vi "Target - REF - MAIN.vi"() -> ()   [LabVIEW 2013]
doc: "This VI first configures the sample clock on the module and starts it. Then it acquires single point data from four channels. In order for the loop rate to be synchronized with the module's clock, the data is pipelined before it is written it to a DMA FIFO so it can be transfered to the host."
uses:
  <vilib>/LabVIEW Targets/FPGA/cRIO/shared/nicrio_ModuleControls/nicrio_cRIO-9234_DataRatesRing2.ctl
  <vilib>/rvi/eio/common/nirviEmuTemplatePropertySet_errors.vi
  <vilib>/rvi/eio/common/nirviEmuTemplateMethod_errors.vi
  <vilib>/rvi/Emulation/niFpgaSctlEmulationGetInTimedLoop.vi
  <vilib>/rvi/Emulation/niFpgaEmulationReportErrorSimple.vi
  <vilib>/rvi/Emulation/niFpgaGetClockAttributes.vi
  <vilib>/rvi/Emulation/niFpgaCriticalErrorInLSC.vi
  <vilib>/rvi/eio/common/nirviEmuTemplatePropertyGet_noerrors.vi
  <vilib>/rvi/interface/RandomDataEmulation/nirviRandomDataFPGAFIFO.vi
  <vilib>/rvi/interface/RandomDataEmulation/niFpgaRandomDataHandleErrors.vi
  <vilib>/eio/EIOPropertyNode/EIOPropertyNode.xnode
  <vilib>/eio/EIONode/EIONode.xnode
  <vilib>/eio/EIOMethodNode/EIOMethodNode.xnode
  <vilib>/rvi/DataTransferAndStorage/Container/XNode/niFpgaContainer.xnode
  <vilib>/rvi/interface/RandomDataEmulation/nirviRandomDataFpgaReadWriteTemplate.vi
  <vilib>/rvi/eio/common/nirviEmuTemplatePropertyGet_errors.vi
  <vilib>/rvi/eio/common/nirviEmuTemplatePropertySet_noerrors.vi
  GPS Timekeeper Files/FPGA Timekeeper.lvlib
panel:
  out "FPGA Timekeeper time (ns)":u64
  out "GPS status":T1(ring)
  out "FPGA Timekeeper locked":bool
  out "offset from time reference":i32
  out "antenna status":T2(ring)
  out "satellites available":u8
  out "UTC offset":i8
  out "UTC offset valid":bool
  in  "Data Rate":T3=1 items=["51.200 kS/s (NI 9234)"=1, "25.600 kS/s (NI 9234)"=2, "17.067 kS/s (NI 9234)"=3, "12.800 kS/s (NI 9234)"=4, "10.240 kS/s (NI 9234)"=5, "8.533 kS/s (NI 9234)"=6, "7.314 kS/s (NI 9234)"=7, "6.400 kS/s (NI 9234)"=8, "5.689 kS/s (NI 9234)"=9, "5.120 kS/s (NI 9234)"=10, "4.654 kS/s (NI 9234)"=11, "4.267 kS/s (NI 9234)"=12, "3.938 kS/s (NI 9234)"=13, "3.657 kS/s (NI 9234)"=14, "3.413 kS/s (NI 9234)"=15, "3.200 kS/s (NI 9234)"=16, "3.012 kS/s (NI 9234)"=17, "2.845 kS/s (NI 9234)"=18, "2.695 kS/s (NI 9234)"=19, "2.560 kS/s (NI 9234)"=20, "2.438 kS/s (NI 9234)"=21, "2.328 kS/s (NI 9234)"=22, "2.226 kS/s (NI 9234)"=23, "2.133 kS/s (NI 9234)"=24, "2.048 kS/s (NI 9234)"=25, "1.969 kS/s (NI 9234)"=26, "1.896 kS/s (NI 9234)"=27, "1.829 kS/s (NI 9234)"=28, "1.765 kS/s (NI 9234)"=29, "1.707 kS/s (NI 9234)"=30, "1.652 kS/s (NI 9234)"=31]
  out "Acq Loop Ticks":u32
  out "FPGA Error":errorcluster
  out "Module Underflow":bool
  out "DMA FIFO Full":bool
  in  "Stop":bool
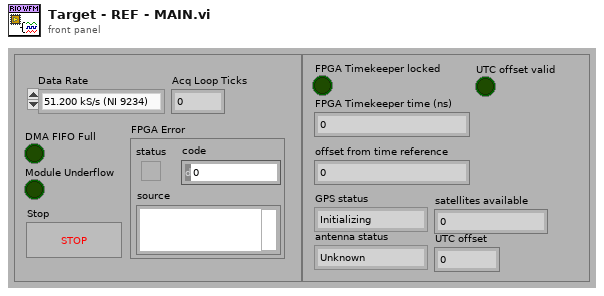
[diagram p1: front panel]
types:
  T1 = enum8{"Initializing", "Normal", "Unable to get fix"}
  T2 = enum8{"Unknown", "Normal", "Absent", "Overcurrent"}
  T3 = typedef "nicrio_cRIO-9234_DataRatesRing2.ctl" = u8
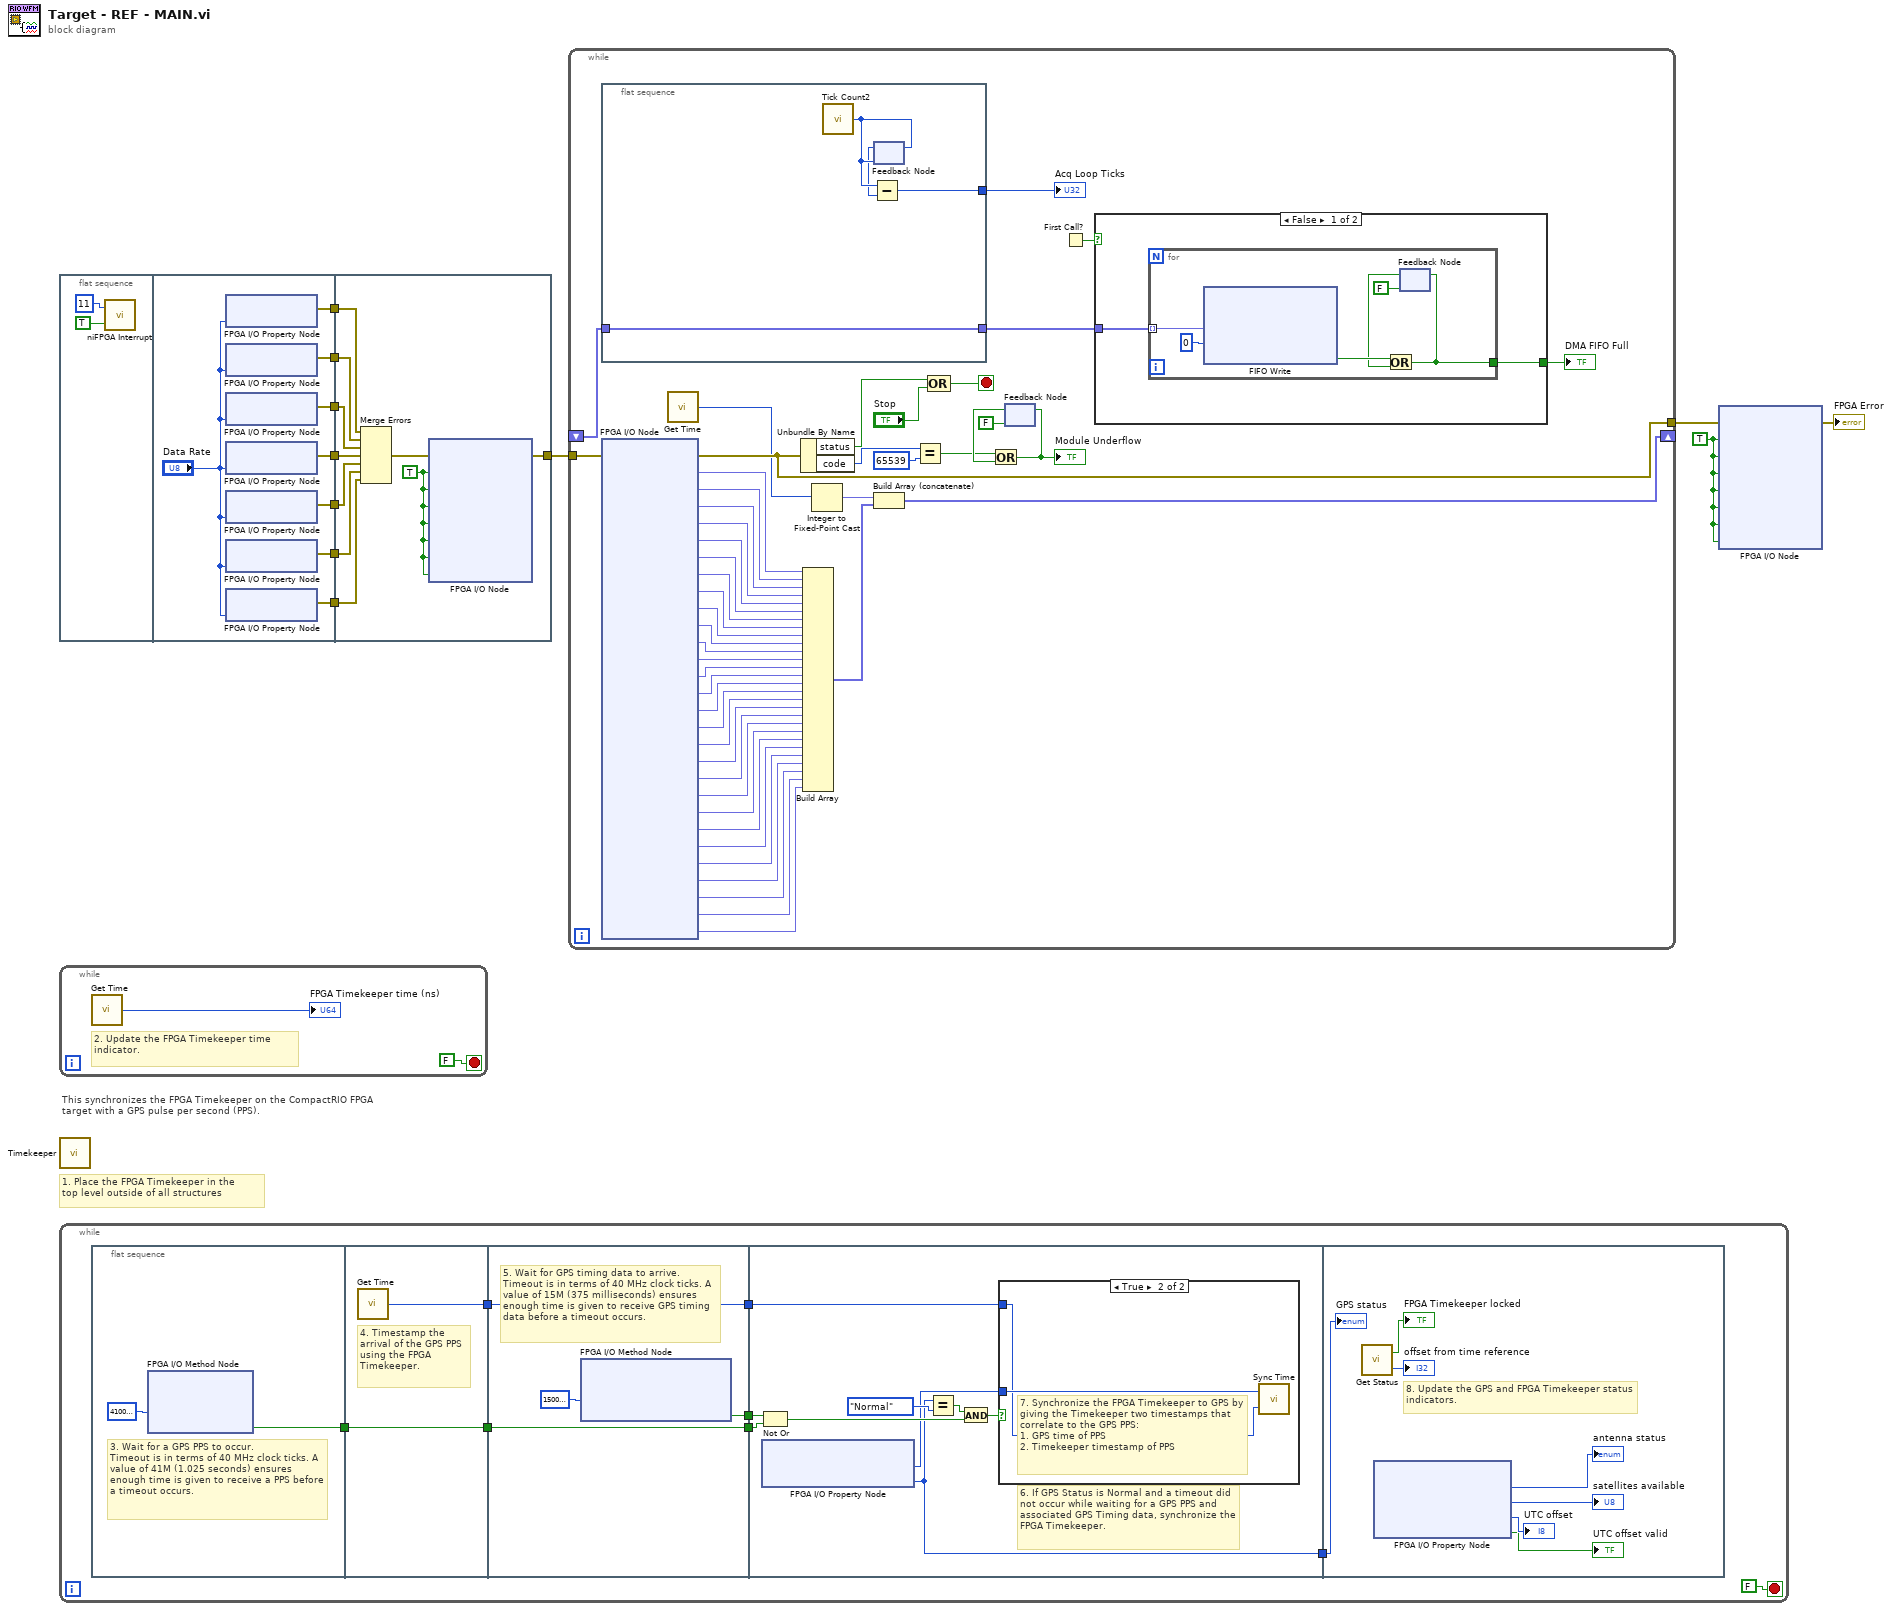
[diagram p0: block diagram]
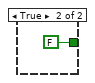
[diagram p3: hidden frame]
diagram:
  w1 = TRUE ("Mod1/Stop")
  # "This synchronizes the FPGA Timekeeper on the CompactRIO FPGA target with a GPS pulse per second (PPS)."
  # "1. Place the FPGA Timekeeper in the\ntop level outside of all structures"
  n1 = flat-sequence {
    tunnel: [w21] -> w10
    tunnel: [w20] -> w9
    tunnel: [w19] -> w6
    tunnel: [w18] -> w5
    tunnel: [w16] -> w4
    tunnel: [w15] -> w3
    tunnel: [w14] -> w2
    tunnel: [w31] -> w11
    tunnel: w10 -> [w29]
    tunnel: w9 -> [w28]
    tunnel: w6 -> [w27]
    tunnel: w5 -> [w26]
    tunnel: w4 -> [w25]
    tunnel: w3 -> [w24]
    tunnel: w2 -> [w23]
    frame #0 {
      n2 = call <vilib>:"niFPGA Interrupt.vi"("Wait Until Cleared (F)"=TRUE ("Wait Until Cleared"), "IRQ Number (0)"=u8 11 ("IRQ Number")) -> ()  [unwired: 1 in]
    }
    frame #1 {
      n3 = xnode "FPGA I/O Property Node"("Data Rate"="Data Rate") -> ("error out"=w21:errorcluster)  [unwired: 2 in, 1 out]
      n4 = xnode "FPGA I/O Property Node"("Data Rate"="Data Rate") -> ("error out"=w20:errorcluster)  [unwired: 2 in, 1 out]
      n5 = xnode "FPGA I/O Property Node"("Data Rate"="Data Rate") -> ("error out"=w19:errorcluster)  [unwired: 2 in, 1 out]
      n6 = xnode "FPGA I/O Property Node"("Data Rate"="Data Rate") -> ("error out"=w18:errorcluster)  [unwired: 2 in, 1 out]
      n7 = xnode "FPGA I/O Property Node"("Data Rate"="Data Rate") -> ("error out"=w16:errorcluster)  [unwired: 2 in, 1 out]
      n8 = xnode "FPGA I/O Property Node"("Data Rate"="Data Rate") -> ("error out"=w15:errorcluster)  [unwired: 2 in, 1 out]
      n9 = xnode "FPGA I/O Property Node"("Data Rate"="Data Rate") -> ("error out"=w14:errorcluster)  [unwired: 2 in, 1 out]
    }
    frame #2 {
      w22 = TRUE ("Mod1/Start")
      n10 = Merge Errors(w29, w28, w27, w26, w25, w24, w23) -> (w30:errorcluster)
      n11 = xnode "FPGA I/O Node"("error in"=w30, "Mod1/Start"=w22, "Mod2/Start"=w22, "Mod3/Start"=w22, "Mod4/Start"=w22, "Mod5/Start"=w22, "Mod6/Start"=w22, "Mod7/Start"=w22) -> ("error out"=w31:errorcluster)  [unwired: 7 in, 7 out]
    }
  }
  n12 = while {
    stop <- FALSE stop-if-true
    # "2. Update the FPGA Timekeeper time indicator."
    n13 = call "Get Time.vi"() -> ("time (ns)"=→"FPGA Timekeeper time (ns)":u64)  [unwired: 1 in]
  }
  n14 = call "Timekeeper.vi"() -> ()  [unwired: 12 in]
  n15 = while {
    stop <- FALSE stop-if-true
    n16 = flat-sequence {
      tunnel: [w42] -> w40
      tunnel: w40 -> [w45]
      tunnel: [w45] -> w39
      tunnel: [w44] -> w37
      tunnel: [w48] -> w41
      tunnel: w39 -> [w47]
      tunnel: [w47] -> w38
      tunnel: w37 -> [w46]
      tunnel: [w46] -> w36
      tunnel: w41 -> [w57]
      tunnel: w38 -> [w56]
      tunnel: w36 -> [w51]
      tunnel: [w50] -> w35
      tunnel: w35 -> [w67]
      frame #0 {
        # "3. Wait for a GPS PPS to occur.\nTimeout is in terms of 40 MHz clock ticks. A value of 41M (1.025 seconds) ensures enough time is given to receive a PPS before a timeout occurs."
        n17 = xnode "FPGA I/O Method Node"("Timeout"=41000000) -> ("Timed Out"=w42:bool)  [unwired: 1 in, 1 out]
      }
      frame #1 {
        # "4. Timestamp the arrival of the GPS PPS using the FPGA Timekeeper."
        n18 = call "Get Time.vi"() -> ("time (ns)"=w44:u64)  [unwired: 1 in]
      }
      frame #2 {
        # "5. Wait for GPS timing data to arrive.\nTimeout is in terms of 40 MHz clock ticks. A value of 15M (375 milliseconds) ensures enough time is given to receive GPS timing data before a timeout occurs."
        n19 = xnode "FPGA I/O Method Node"("Timeout"=15000000) -> ("Timed Out"=w48:bool)  [unwired: 1 in, 1 out]
      }
      frame #3 {
        # "6. If GPS Status is Normal and a timeout did not occur while waiting for a GPS PPS and associated GPS Timing data, synchronize the FPGA Timekeeper."
        n20 = Not Or(1:w56, 2:w57) -> (0:w54:bool)
        n21 = xnode "FPGA I/O Property Node"() -> ("PPS Timestamp (TAI)"=w52:u64, "GPS Status"=w50:T1)  [unwired: 1 in, 1 out]
        n22 = Equal?(x=w50, y=T1."Normal") -> (x = y?=w55:bool)
        n23 = And(x=w55, y=w54) -> (x .and. y?=w53:bool)
        n24 = case shown="True" w53 {
          tunnel: w52 -> [_ w60]
          tunnel: w51 -> [_ w59]
          frame False {
          }
          frame True {
            # "7. Synchronize the FPGA Timekeeper to GPS by giving the Timekeeper two timestamps that correlate to the GPS PPS:\n1. GPS time of PPS\n2. Timekeeper timestamp of PPS"
            n25 = call "Sync Time.vi"("FPGA Timekeeper time (ns)"=w59, "time reference time (ns)"=w60) -> ()
          }
        }
      }
      frame #4 {
        # "8. Update the GPS and FPGA Timekeeper status indicators."
        n26 = call "Get Status.vi"() -> ("FPGA Timekeeper locked"=→"FPGA Timekeeper locked":bool, "offset from time reference"=→"offset from time reference":i32)
        n27 = xnode "FPGA I/O Property Node"() -> ("Antenna Status"=→"antenna status":T2, "Satellites Available"=→"satellites available":u8, "UTC Offset"=→"UTC offset":i8, "UTC Offset Valid"=→"UTC offset valid":bool)  [unwired: 1 in, 1 out]
        "GPS status" <- w67
      }
    }
  }
  n28 = while {
    tunnel: [w111] -> w8
    shift-right: [w99] -> _
    shift-left: _ -> [w107]
    tunnel: w11 -> [w100]
    stop <- w114 stop-if-true
    n29 = flat-sequence {
      tunnel: [w126] -> w109
      tunnel: w107 -> [w125]
      tunnel: [w125] -> w108
      frame #0 {
        n30 = call "Tick Count2"() -> ("Tick Count(Ticks)"=w128:u32)
        n31 = feedback-in #1(w128) -> ()
        n32 = feedback #1(w128) -> (w127:u32)
        n33 = Subtract(x=w128, y=w127) -> (x-y=w126:u32)
      }
    }
    n34 = xnode "FPGA I/O Node"("error in"=w100) -> ("error out"=w111:errorcluster, "Mod1/AI0"=w96:fxp<+/-,24,4>, "Mod1/AI1"=w95:fxp<+/-,24,4>, "Mod1/AI2"=w94:fxp<+/-,24,4>, "Mod1/AI3"=w93:fxp<+/-,24,4>, "Mod2/AI0"=w92:fxp<+/-,24,4>, "Mod2/AI1"=w91:fxp<+/-,24,4>, "Mod2/AI2"=w90:fxp<+/-,24,4>, "Mod2/AI3"=w89:fxp<+/-,24,4>, "Mod3/AI0"=w88:fxp<+/-,24,4>, "Mod3/AI1"=w87:fxp<+/-,24,4>, "Mod3/AI2"=w86:fxp<+/-,24,4>, "Mod3/AI3"=w85:fxp<+/-,24,4>, "Mod4/AI0"=w84:fxp<+/-,24,4>, "Mod4/AI1"=w83:fxp<+/-,24,4>, "Mod4/AI2"=w82:fxp<+/-,24,4>, "Mod4/AI3"=w81:fxp<+/-,24,4>, "Mod5/AI0"=w79:fxp<+/-,24,4>, "Mod5/AI1"=w78:fxp<+/-,24,4>, "Mod5/AI2"=w77:fxp<+/-,24,4>, "Mod5/AI3"=w76:fxp<+/-,24,4>, "Mod6/AI0"=w75:fxp<+/-,24,4>, "Mod6/AI1"=w74:fxp<+/-,24,4>, "Mod6/AI2"=w73:fxp<+/-,24,4>, "Mod6/AI3"=w72:fxp<+/-,24,4>, "Mod7/AI0"=w71:fxp<+/-,24,4>, "Mod7/AI1"=w70:fxp<+/-,24,4>, "Mod7/AI2"=w69:fxp<+/-,24,4>, "Mod7/AI3"=w68:fxp<+/-,24,4>)  [unwired: 28 in, 28 out]
    n35 = call "Get Time.vi"() -> ("time (ns)"=w80:u64)  [unwired: 1 in]
    n36 = Unbundle By Name(w111) -> ("status"=w106:bool, "code"=w112:i32)
    n37 = Build Array(w96, w95, w94, w93, w92, w91, w90, w89, w88, w87, w86, w85, w84, w83, w82, w81, w79, w78, w77, w76, w75, w74, w73, w72, w71, w70, w69, w68) -> (w97:fxp<+/-,24,4>[])
    n38 = Integer to Fixed-Point Cast(integer=w80) -> (fixed-point=w98:fxp<+/-,64,44>)  [unwired: 1 in]
    n39 = Build Array (concatenate)(w98, w97) -> (w99:fxp<+/-,64,44>[])
    n40 = Equal?(x=w112, y=65539) -> (x = y?=w103:bool)
    n41 = Compound Arithmetic op=OR(w106, "Stop") -> (w114:bool)
    n42 = feedback #2(FALSE) -> (w105:bool)
    n43 = Or(x=w103, y=w105) -> (x .or. y?=w102:bool)
    "Module Underflow" <- w102
    n44 = feedback-in #2(w102) -> ()
    n45 = First Call?() -> (First Call?: T/F=w101:bool)
    n46 = case shown="False" w101 {
      tunnel: [w117 FALSE] -> w110
      tunnel: w108 -> [w116 _]
      frame False {
        n47 = for {
          tunnel: [w120] -> w117
          tunnel: w116 -> [w118] mode=indexing
          n48 = xnode ("FIFO Write")("Element"=w118, "Timeout"=0) -> ("Timed Out?"=w123:bool)  [unwired: 1 in, 1 out]
          n49 = feedback #3(FALSE) -> (w121:bool)
          n50 = Or(x=w123, y=w121) -> (x .or. y?=w120:bool)
          n51 = feedback-in #3(w120) -> ()
        }
      }
      frame True {
      }
    }
    "DMA FIFO Full" <- w110
    "Acq Loop Ticks" <- w109
  }
  n52 = xnode "FPGA I/O Node"("error in"=w8, "Mod1/Stop"=w1, "Mod2/Stop"=w1, "Mod3/Stop"=w1, "Mod4/Stop"=w1, "Mod5/Stop"=w1, "Mod6/Stop"=w1, "Mod7/Stop"=w1) -> ("error out"=→"FPGA Error":errorcluster)  [unwired: 7 in, 7 out]
